vi "NI_FPGA_PPG.pdc handler.vi"(0 "i ref in":refnum<vi>, 3 "ms timeout (10000)":i32=10000, 5 "error in (no error)":errorcluster) -> (14 "i ref out":refnum<vi>, 17 "timed out":bool, 19 "error out":errorcluster)   [LabVIEW 2014, in "NI_FPGA_PPG.lvlib"]
doc: "Checks FPGA status, updates DIM services and disables periodic polling after specified standby time (if device status != run).\n\nLicense Agreement for this software:\n\nCopyright (C) 2009\nFalk Ziegler\nInstitut für Physik\nErnst-Moritz-Arndt Universität\nFelix-Hausdorff-Str. 6\n17487 Greifswald\n\nContact: Falk Ziegler, ziegler@physik.uni-greifswald.de\n\nThis program is free software: you can redistribute it and/or modify it under the terms of the GNU General Public License as published by the Free Software Foundation, either version 3 of the License, or (at your option) any later version.\n\nThis program is distributed in the hope that it will be useful, but WITHOUT ANY WARRANTY; without even the implied warranty of MERCHANTABILITY or FITNESS FOR A PARTICULAR PURPOSE. See the GNU General Public License for more details.\n\nYou should have received a copy of the GNU General Public License along with this program. If not, see <http://www.gnu.org/licenses/>.\n\nFor all questions and ideas contact: ziegler@physik.uni-greifswald.de or d.beck@gsi.de\nLast update: 01-Sep-2009"
uses:
  NI_FPGA_PPG.lvlib
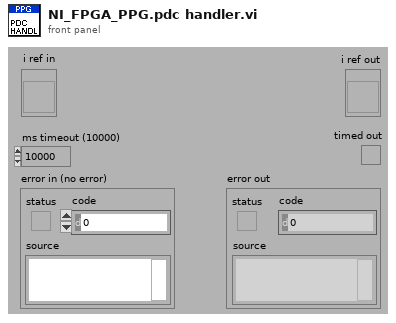
[diagram p1: front panel]
types:
  T1 = typedef "NI_FPGA_PPG.lvlib/NI_FPGA_PPG.i attribute.ctl" = cluster{"dim_service_id":cluster{"dim_actual_device_status":i32, "dim_event_data":i32, "dim_cmd_data":i32, "dim_cmd_data _description":i32, "dim_channel_description":i32}, "VISA":refnum<visa-resource-name>, "actual_device_status":i32, "event_data_id":i32, "pdc_enabled":bool, "pdc_timestamp":u32, "cmd_data_string":string, "cmd_data_size":i32, "cmd_data_description_string":string, "cmd_data_description_size":i32, "channel_description_string":string, "channel_description_size":i32}
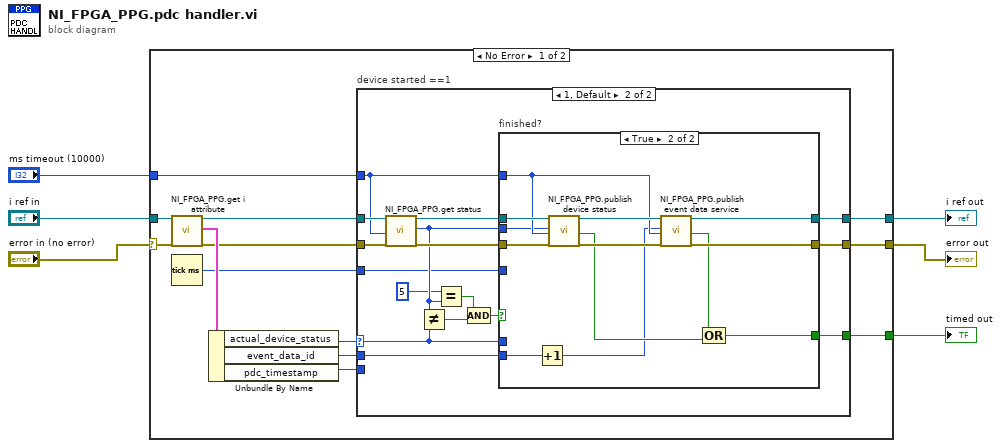
[diagram p0: block diagram]
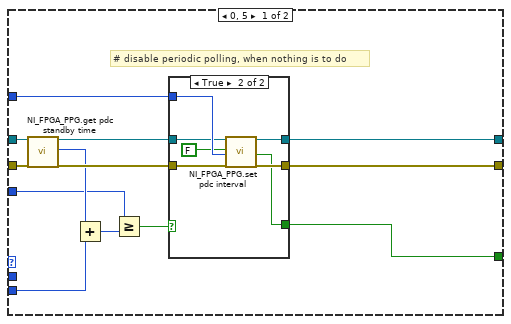
[diagram p2: hidden frame]
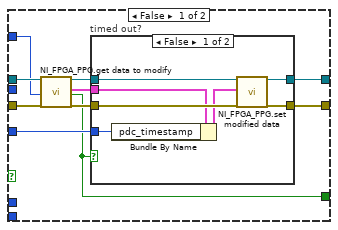
[diagram p4: hidden frame]
diagram:
  n1 = case shown="No Error" "error in (no error)" {
    selector: "error in (no error)" -> [w18 w90]
    tunnel: "i ref in" -> [w19 w91]
    tunnel: [w13 w91] -> w4
    tunnel: [w12 w90] -> w3
    tunnel: "ms timeout (10000)" -> [w14 _]
    tunnel: [w9 _] -> w1
    frame No Error {
      n2 = call "NI_FPGA_PPG.get i attribute.vi"("i ref in"=w19, "error in (no error)"=w18) -> ("i ref out"=w16:refnum<vi>, "i attribute"=w17:T1, "error out"=w15:errorcluster)  [unwired: 15 in]
      n3 = Tick Count (ms)() -> (millisecond timer value=w7:u32)
      n4 = Unbundle By Name(w17) -> ("actual_device_status"=w8:i32, "event_data_id"=w11:i32, "pdc_timestamp"=w10:u32)
      n5 = case "device started ==1" shown="1, Default" w8 {
        selector: w8 -> [_ w46]
        tunnel: w16 -> [w27 w57]
        tunnel: w15 -> [w26 w56]
        tunnel: w14 -> [w31 w52]
        tunnel: [w30 w49] -> w13
        tunnel: [w29 w48] -> w12
        tunnel: w11 -> [_ w45]
        tunnel: w10 -> [w25 _]
        tunnel: [w28 w47] -> w9
        tunnel: w7 -> [w20 w43]
        frame 0, 5 {
          # "# disable periodic polling, when nothing is to do"
          n6 = call "NI_FPGA_PPG.get pdc standby time.vi"("i ref in"=w27, "error in (no error)"=w26) -> ("i ref out"=w24:refnum<vi>, "pdc_standby"=w22:i32, "error out"=w23:errorcluster)  [unwired: 15 in]
          n7 = Add(x=w22, y=w25) -> (x+y=w32:u32)
          n8 = Greater Or Equal?(x=w20, y=w32) -> (x >= y?=w21:bool)
          n9 = case shown="True" w21 {
            tunnel: w31 -> [_ w41]
            tunnel: [w34 w40] -> w30
            tunnel: [w33 w39] -> w29
            tunnel: [_ w38] -> w28
            tunnel: w24 -> [w34 w37]
            tunnel: w23 -> [w33 w36]
            frame False {
            }
            frame True {
              n10 = call "NI_FPGA_PPG.set pdc interval.vi"("i ref in"=w37, "enable_pdc"=FALSE, "ms timeout (10000)"=w41, "error in (no error)"=w36) -> ("i ref out"=w40:refnum<vi>, "timed out"=w38:bool, "error out"=w39:errorcluster)  [unwired: 13 in]
            }
          }
        }
        frame 1, Default {
          n11 = call "NI_FPGA_PPG.get status.vi"("i ref in"=w57, "ms timeout (10000)"=w52, "error in (no error)"=w56) -> ("i ref out"=w51:refnum<vi>, "FPGA_status"=w44:i32, "error out"=w50:errorcluster)  [unwired: 13 in, 1 out]
          n12 = Not Equal?(x=w44, y=w46) -> (x != y?=w54:bool)
          n13 = Equal?(x=5, y=w44) -> (x = y?=w55:bool)
          n14 = Compound Arithmetic op=AND(w55, w54) -> (w53:bool)
          n15 = case "finished?" shown="True" w53 {
            tunnel: w51 -> [w67 w89]
            tunnel: w50 -> [w66 w88]
            tunnel: w52 -> [w65 w85]
            tunnel: [w61 w84] -> w49
            tunnel: [w62 w83] -> w48
            tunnel: w46 -> [_ _]
            tunnel: [w58 w80] -> w47
            tunnel: w45 -> [_ w79]
            tunnel: w44 -> [_ w78]
            tunnel: w43 -> [w59 _]
            frame False {
              n16 = call "NI_FPGA_PPG.get data to modify.vi"("i ref in"=w67, "ms timeout (10000)"=w65, "error in (no error)"=w66) -> ("i ref out"=w63:refnum<vi>, "i attribute"=w60:T1, "timed out"=w58:bool, "error out"=w64:errorcluster)  [unwired: 13 in]
              n17 = case "timed out?" shown="False" w58 {
                tunnel: w64 -> [w73 w75]
                tunnel: w63 -> [w74 w76]
                tunnel: [w72 w75] -> w62
                tunnel: [w71 w76] -> w61
                tunnel: w60 -> [w70 _]
                tunnel: w59 -> [w68 _]
                frame False {
                  n18 = Bundle By Name(cluster=w70, "pdc_timestamp"=w68) -> (w69:T1)
                  n19 = call "NI_FPGA_PPG.set modified data.vi"("i ref in"=w74, "i attribute"=w69, "error in (no error)"=w73) -> ("i ref out"=w71:refnum<vi>, "error out"=w72:errorcluster)  [unwired: 15 in]
                }
                frame True {
                }
              }
            }
            frame True {
              n20 = Increment(x=w79) -> (x+1=w77:i32)
              n21 = call "NI_FPGA_PPG.publish device status.vi"("i ref in"=w89, "actual_status"=w78, "ms timeout (10000)"=w85, "error in (no error)"=w88) -> ("i ref out"=w87:refnum<vi>, "timed out"=w82:bool, "error out"=w86:errorcluster)  [unwired: 13 in]
              n22 = call "NI_FPGA_PPG.publish event data service.vi"("i ref in"=w87, "event_data_id"=w77, "ms timeout (10000)"=w85, "error in (no error)"=w86) -> ("i ref out"=w84:refnum<vi>, "timed out"=w81:bool, "error out"=w83:errorcluster)  [unwired: 13 in]
              n23 = Compound Arithmetic op=OR(w81, w82) -> (w80:bool)
            }
          }
        }
      }
    }
    frame Error {
    }
  }
  "error out" <- w3
  "i ref out" <- w4
  "timed out" <- w1
